vi "SelectClassWire.vi"() -> ()   [LabVIEW 2020]
uses:
  <resource>/Framework/Providers/Open_GDS/ClassProviders/Provider_BaseClassInterface/BaseProvider_SubVIs/BaseProvider_WireList.ctl
  <resource>/Framework/Providers/Open_GDS/ClassProviders/Provider_BaseClassInterface/BaseProvider_SubVIs/BaseProvider_WireStyleType.ctl
  <vilib>/Utility/miscctls.llb/LVPositionTypeDef.ctl
  8146e3c4-7363-43e9-93da-efe32bb20ee4.vi
  c84afe10-fc65-4d8b-b200-0de5f07e0a9c.vi
panel:
  in  "WireSelectionList":T1
  out "Wire Style":cluster{"Name":string, "Wire":picture}
  out "WireStyleSelected":string
  in  "error in (no error)":errorcluster
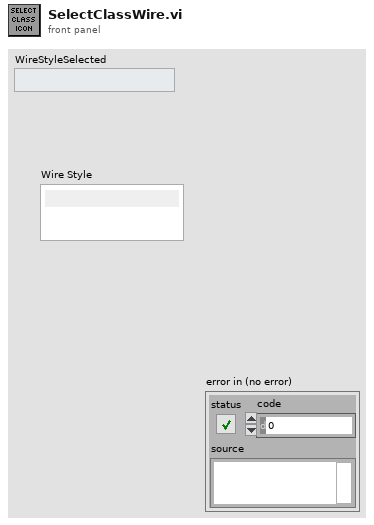
[diagram p1: front panel]
types:
  T1 = typedef "BaseProvider_WireList.ctl" = cluster{"WireStyle":T2[], "WireEditor":bool}
  T2 = typedef "BaseProvider_WireStyleType.ctl" = cluster{"Boolean":bool, "Wire":picture, "Name":string, "Status":u16}
  T3 = typedef "LVPositionTypeDef.ctl" = cluster{"Left":i32, "Top":i32}
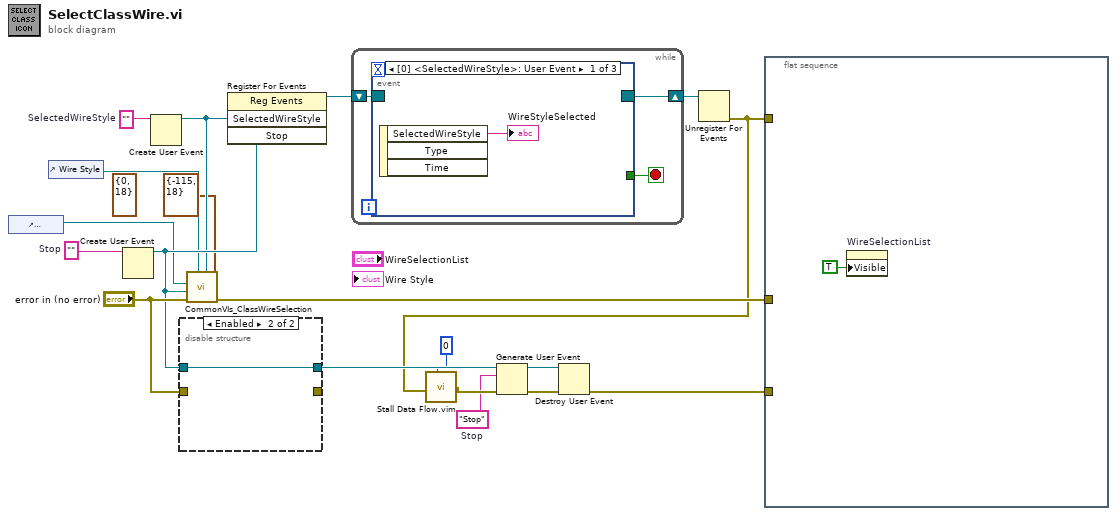
[diagram p0: block diagram]
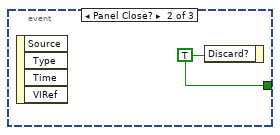
[diagram p2: hidden frame]
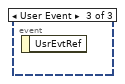
[diagram p3: hidden frame]
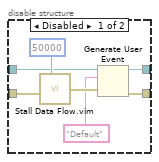
[diagram p4: hidden frame]
diagram:
  (unwired) T3 {"Left"=0, "Top"=18} ("Offset(-300,0)")
  w12 = ""  # SelectedWireStyle
  w13 = "Stop"  # Stop
  w18 = ""  # Stop
  n1 = control-ref of="WireSelectionList"() -> (w5:refnum<vi>)
  n2 = control-ref of="Wire Style"() -> (w6:refnum<vi>)
  n3 = Create User Event(user event datatype=w18) -> (user event=w10:refnum<user-event>)  [unwired: 1 in, 1 out]
  n4 = Create User Event(user event datatype=w12) -> (user event=w9:refnum<user-event>)  [unwired: 1 in, 1 out]
  n5 = disable-structure shown="Enabled" {
    disable-tunnel: "error in (no error)" -> [w26 _]
    disable-tunnel: [w24 _] -> _
    disable-tunnel: [w23 w27] -> w16
    disable-tunnel: w10 -> [w20 w27]
    frame Disabled {
      n6 = call "Stall Data Flow.vim"("value in"=w26, "milliseconds to wait"=u32 50000) -> ("value out"=w25:errorcluster)  [unwired: 1 out]
      n7 = Generate User Event(user event=w20, event data cluster="Default", error in=w25) -> (user event out=w23:refnum<user-event>, error out=w24:errorcluster)  [unwired: 1 in]
    }
    frame Enabled {
    }
  }
  n8 = call <resource>:"CommonVIs_ClassWireSelection.vi"("Offset(-300,0)"=T3 {"Left"=-115, "Top"=18}, "WireStyleSelected"=w9, "SelectedWireStyle"=w6, "error in (no error)"="error in (no error)", "Messages(Stop or Empty string will stop this VI)"=w10, "WireSelectionList"=w5) -> ("error out"=w3:errorcluster)  [unwired: 5 in]
  n9 = register-events(w9, w10) -> (reference out=w11:refnum<event-registration>)  [unwired: 2 in, 1 out]
  n10 = while {
    shift-right: [w29] -> w8
    shift-left: w11 -> [w30]
    stop <- w28 stop-if-true
    n11 = event shown="[0] <SelectedWireStyle>: User Event" {
      selector: w30 -> [_ _ _]
      dyn-events: [_ _ _] -> w29
      timeout: _ -> [_ _ _]
      tunnel: [_ w32 _] -> w28
      event User Event {
        n12 = event-data() -> ("SelectedWireStyle"=→"WireStyleSelected":string)  [unwired: 1 in, 2 out]
      }
      event Panel Close? {
        w32 = TRUE ("Discard?")
        n13 = event-data() -> ()  [unwired: 1 in, 4 out]
        n14 = event-data("Discard?"=w32) -> ()  [unwired: 1 in, 1 out]
      }
      event User Event {
        n15 = event-data() -> ()  [unwired: 1 in, 1 out]
      }
    }
  }
  n16 = Unregister For Events(event registration refnum=w8) -> (error out=w1:errorcluster)  [unwired: 1 in]
  n17 = call "Stall Data Flow.vim"("value in"=w1, "milliseconds to wait"=u32 0) -> ("value out"=w17:errorcluster)  [unwired: 1 out]
  n18 = Generate User Event(user event=w16, event data cluster=w13, error in=w17) -> (user event out=w15:refnum<user-event>, error out=w14:errorcluster)  [unwired: 1 in]
  n19 = Destroy User Event(user event=w15, error in=w14) -> (error out=w4:errorcluster)
  n20 = flat-sequence {
    tunnel: w1 -> [_]
    tunnel: w4 -> [_]
    tunnel: w3 -> [_]
    frame #0 {
      n21 = property on="WireSelectionList" class="Clust (strict)"("Visible"=TRUE) -> ()  [unwired: 2 in, 2 out]
    }
  }
